vi "Load Test Double.vi"(11 "Parameterized Test Case Test in":refnum<class "Parameterized Test Case Test.lvclass">) -> (0 "error out":errorcluster, 3 "Parameterized Test Case out":refnum<class "Parameterized Test Case.lvclass">)   [LabVIEW 2020, in "Parameterized Test Case Test.lvclass"]
uses:
  Parameterized Test Case Test.lvclass
  source/Parameterized Test Case/Parameterized Test Case.lvclass
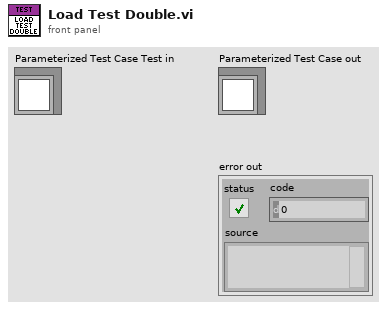
[diagram p1: front panel]
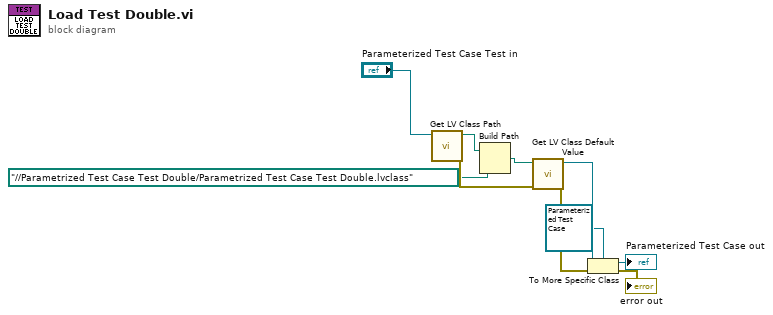
[diagram p0: block diagram]
diagram:
  n1 = call <vilib>:"Get LV Class Path.vi"("object"="Parameterized Test Case Test in") -> ("error out"=w9:errorcluster, "class path"=w4:path)  [unwired: 9 in]
  n2 = Build Path(base path=w4, name or relative path=path "../../Parametrized Test Case Test Double/Parametrized Test Case Test Double.lvclass" ("class path")) -> (appended path=w6:path)
  n3 = call <vilib>:"Get LV Class Default Value.vi"("error in (no error)"=w9, "class path"=w6) -> ("error out"=w8:errorcluster, "object"=w7:refnum<class>)  [unwired: 8 in]
  n4 = To More Specific Class(target class=refnum<class "Parameterized Test Case.lvclass"> refnum ("Parameterized Test Case.lvclass"), reference=w7, error in=w8) -> (specific class reference=→"Parameterized Test Case out":refnum<class "Parameterized Test Case.lvclass">, error out=→"error out":errorcluster)
